vi "NI5112.ProcEvents.vi"(0 "i ref in":refnum<vi>, 5 "error in":errorcluster) -> (14 "i ref out":refnum<vi>, 19 "error out":errorcluster)   [LabVIEW 2014, in "NI5112.lvlib"]
doc: "This method is used to define the events the object will listen to. Add your own events here."
uses:
  NI5112.lvlib
  CS_Core/BaseProcess/BaseProcess.event definition.ctl
  CS_Core/CAEObj/CAEObj.event definition.ctl
  CS_Core/BaseProcess/BaseProcess.descriptor string definition.ctl
  CS_Core/BaseProcess/BaseProcess.lvlib
  CS_Core/CAEObj/CAEObj.lvlib
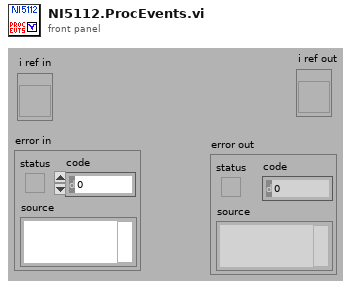
[diagram p1: front panel]
types:
  T1 = typedef "BaseProcess.lvlib/BaseProcess.event definition.ctl" = cluster{"CAEEvtDef":T2, "Data Descriptor":T3}
  T2 = typedef "CAEObj.lvlib/CAEObj.event definition.ctl" = cluster{"URL":string, "enable":bool, "ignoreResID":bool}
  T3 = typedef "BaseProcess.lvlib/BaseProcess.descriptor string definition.ctl" = string
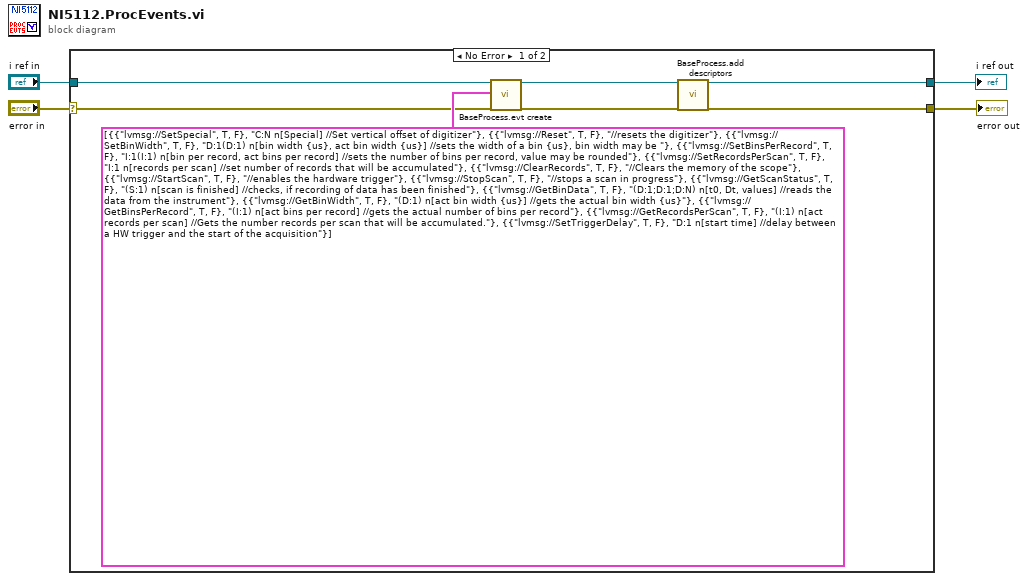
[diagram p0: block diagram]
diagram:
  n1 = case shown="No Error" "error in" {
    selector: "error in" -> [w5 w12]
    tunnel: "i ref in" -> [w11 w13]
    tunnel: [w9 w13] -> w3
    tunnel: [w7 w12] -> w2
    frame No Error {
      n2 = call "BaseProcess.evt create.vi"("i ref in"=w11, "newEvents"=T1[] [{"CAEEvtDef"={"URL"="lvmsg://SetSpecial", "enable"=TRUE, "ignoreResID"=FALSE}, "Data Descriptor"="C:N n[Special] //Set vertical offset of digitizer"}, {"CAEEvtDef"={"URL"="lvmsg://Reset", "enable"=TRUE, "ignoreResID"=FALSE}, "Data Descriptor"="//resets the digitizer"}, {"CAEEvtDef"={"URL"="lvmsg://SetBinWidth", "enable"=TRUE, "ignoreResID"=FALSE}, "Data Descriptor"="D:1(D:1) n[bin width {us}, act bin width {us}] //sets the width of a bin {us}, bin width may be "}, {"CAEEvtDef"={"URL"="lvmsg://SetBinsPerRecord", "enable"=TRUE, "ignoreResID"=FALSE}, "Data Descriptor"="I:1(I:1) n[bin per record, act bins per record] //sets the number of bins per record, value may be rounded"}, {"CAEEvtDef"={"URL"="lvmsg://SetRecordsPerScan", "enable"=TRUE, "ignoreResID"=FALSE}, "Data Descriptor"="I:1 n[records per scan] //set number of records that will be accumulated"}, {"CAEEvtDef"={"URL"="lvmsg://ClearRecords", "enable"=TRUE, "ignoreResID"=FALSE}, "Data Descriptor"="//Clears the memory of the scope"}, {"CAEEvtDef"={"URL"="lvmsg://StartScan", "enable"=TRUE, "ignoreResID"=FALSE}, "Data Descriptor"="//enables the hardware trigger"}, {"CAEEvtDef"={"URL"="lvmsg://StopScan", "enable"=TRUE, "ignoreResID"=FALSE}, "Data Descriptor"="//stops a scan in progress"}, {"CAEEvtDef"={"URL"="lvmsg://GetScanStatus", "enable"=TRUE, "ignoreResID"=FALSE}, "Data Descriptor"="(S:1) n[scan is finished] //checks, if recording of data has been finished"}, {"CAEEvtDef"={"URL"="lvmsg://GetBinData", "enable"=TRUE, "ignoreResID"=FALSE}, "Data Descriptor"="(D:1;D:1;D:N) n[t0, Dt, values] //reads the data from the instrument"}, {"CAEEvtDef"={"URL"="lvmsg://GetBinWidth", "enable"=TRUE, "ignoreResID"=FALSE}, "Data Descriptor"="(D:1) n[act bin width {us}] //gets the actual bin width {us}"}, {"CAEEvtDef"={"URL"="lvmsg://GetBinsPerRecord", "enable"=TRUE, "ignoreResID"=FALSE}, "Data Descriptor"="(I:1) n[act bins per record] //gets the actual number of bins per record"}, {"CAEEvtDef"={"URL"="lvmsg://GetRecordsPerScan", "enable"=TRUE, "ignoreResID"=FALSE}, "Data Descriptor"="(I:1) n[act records per scan] //Gets the number records per scan that will be accumulated."}, {"CAEEvtDef"={"URL"="lvmsg://SetTriggerDelay", "enable"=TRUE, "ignoreResID"=FALSE}, "Data Descriptor"="D:1 n[start time] //delay between a HW trigger and the start of the acquisition"}] ("new events"), "error in (no error)"=w5) -> ("i ref out"=w10:refnum<vi>, "error out"=w8:errorcluster)  [unwired: 13 in, 2 out]
      n3 = call "BaseProcess.add descriptors.vi"("i ref in"=w10, "error in (no error)"=w8) -> ("i ref out"=w9:refnum<vi>, "error out"=w7:errorcluster)  [unwired: 15 in, 1 out]
    }
    frame Error {
    }
  }
  "i ref out" <- w3
  "error out" <- w2
